vi "仁科参数读取.vi"() -> (2 "error out":errorcluster, 3 "簇":T1 {"时间 16"."分钟" format="%.0f分"; "时间 16"."小时" format="%.0f点"; "时间 15"."分钟" format="%.0f分"; "时间 15"."小时" format="%.0f点"; "时间 14"."分钟" format="%.0f分"; "时间 14"."小时" format="%.0f点"; "时间 13"."分钟" format="%.0f分"; "时间 13"."小时" format="%.0f点"; "时间 12"."分钟" format="%.0f分"; "时间 12"."小时" format="%.0f点"; "时间 11"."分钟" format="%.0f分"; "时间 11"."小时" format="%.0f点"; "时间 10"."分钟" format="%.0f分"; "时间 10"."小时" format="%.0f点"; "时间 9"."分钟" format="%.0f分"; "时间 9"."小时" format="%.0f点"; "时间 8"."分钟" format="%.0f分"; "时间 8"."小时" format="%.0f点"; "时间 7"."分钟" format="%.0f分"; "时间 7"."小时" format="%.0f点"; "时间 6"."分钟" format="%.0f分"; "时间 6"."小时" format="%.0f点"; "时间 5"."分钟" format="%.0f分"; "时间 5"."小时" format="%.0f点"; "时间 4"."分钟" format="%.0f分"; "时间 4"."小时" format="%.0f点"; "时间 3"."分钟" format="%.0f分"; "时间 3"."小时" format="%.0f点"; "时间 2"."分钟" format="%.0f分"; "时间 2"."小时" format="%.0f点"; "时间"."分钟" format="%.0f分"; "时间"."小时" format="%.0f点"})   [LabVIEW 2016, in "环境动力监测库.lvlib" / "空调库.lvlib"]
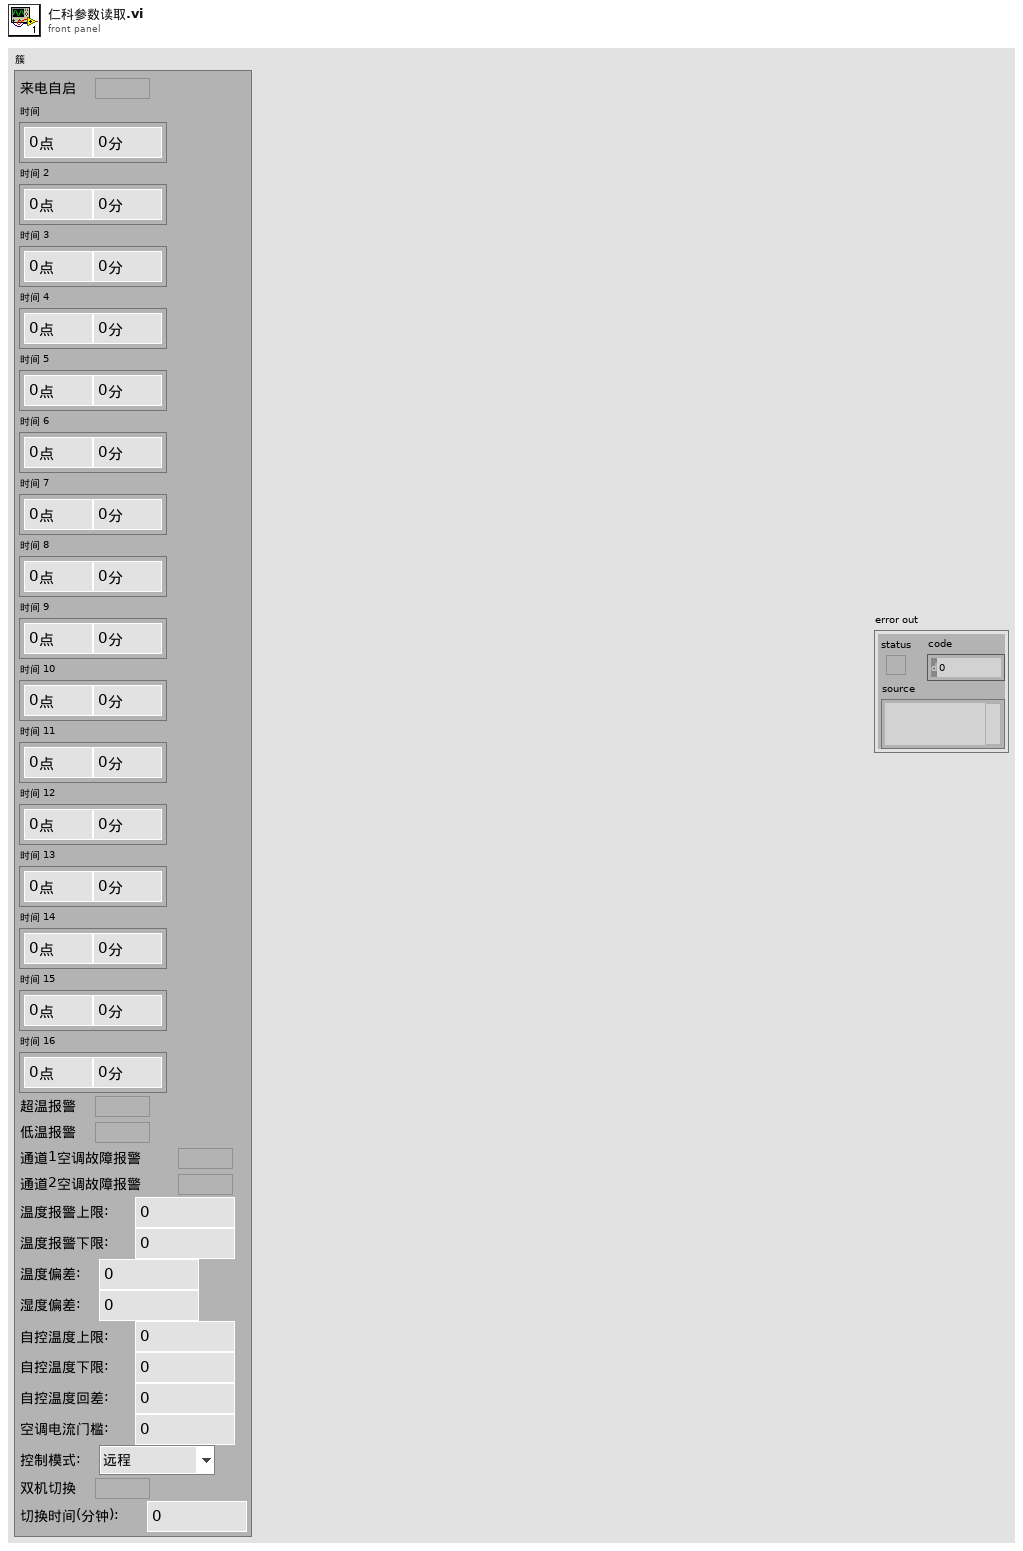
[diagram p1: front panel]
types:
  T1 = cluster{"来电自启":bool, "时间":cluster{"小时":u16, "分钟":u16}, "时间 2":cluster{"小时":u16, "分钟":u16}, "时间 3":cluster{"小时":u16, "分钟":u16}, "时间 4":cluster{"小时":u16, "分钟":u16}, "时间 5":cluster{"小时":u16, "分钟":u16}, "时间 6":cluster{"小时":u16, "分钟":u16}, "时间 7":cluster{"小时":u16, "分钟":u16}, "时间 8":cluster{"小时":u16, "分钟":u16}, "时间 9":cluster{"小时":u16, "分钟":u16}, "时间 10":cluster{"小时":u16, "分钟":u16}, "时间 11":cluster{"小时":u16, "分钟":u16}, "时间 12":cluster{"小时":u16, "分钟":u16}, "时间 13":cluster{"小时":u16, "分钟":u16}, "时间 14":cluster{"小时":u16, "分钟":u16}, "时间 15":cluster{"小时":u16, "分钟":u16}, "时间 16":cluster{"小时":u16, "分钟":u16}, "超温报警":bool, "低温报警":bool, "通道1空调故障报警":bool, "通道2空调故障报警":bool, "温度报警上限:":dbl, "温度报警下限:":dbl, "温度偏差:":dbl, "湿度偏差:":dbl, "自控温度上限:":dbl, "自控温度下限:":dbl, "自控温度回差:":dbl, "空调电流门槛:":dbl, "控制模式:":enum16{"远程", "自动"}, "双机切换":bool, "切换时间(分钟):":dbl}
  T2 = enum16{"open", "read", "write single", "write", "close"}
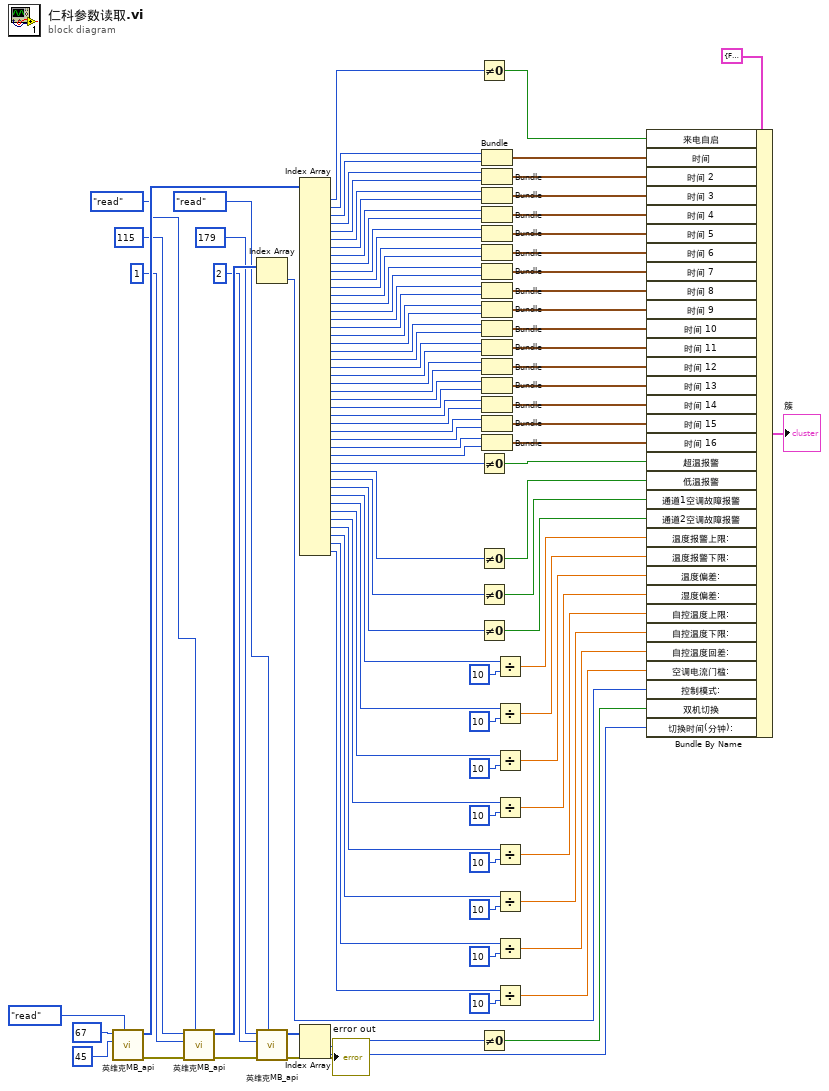
[diagram p0: block diagram]
diagram:
  n1 = call "英维克MB_api.vi"("STEP"=T2."read", "quantity"=u16 45, "starting address"=u16 67) -> ("error out"=w14:errorcluster, "Registers"=w100:u16[])  [unwired: 6 in, 1 out]
  n2 = call "英维克MB_api.vi"("STEP"=T2."read", "Error in"=w14, "quantity"=u16 1, "starting address"=u16 115) -> ("error out"=w7:errorcluster, "Registers"=w13:u16[])  [unwired: 5 in, 1 out]
  n3 = Index Array(array=w13) -> (element=w12:u16)  [unwired: 1 in]
  n4 = call "英维克MB_api.vi"("STEP"=T2."read", "Error in"=w7, "quantity"=u16 2, "starting address"=u16 179) -> ("error out"=→"error out":errorcluster, "Registers"=w11:u16[])  [unwired: 5 in, 1 out]
  n5 = Index Array(array=w100) -> (element #1=w99:u16, element #2=w98:u16, element #3=w97:u16, element #4=w96:u16, element #5=w95:u16, element #6=w91:u16, element #7=w90:u16, element #8=w89:u16, element #9=w88:u16, element #10=w85:u16, element #11=w84:u16, element #12=w83:u16, element #13=w82:u16, element #14=w79:u16, element #15=w78:u16, element #16=w77:u16, element #17=w76:u16, element #18=w75:u16, element #19=w74:u16, element #20=w73:u16, element #21=w72:u16, element #22=w71:u16, element #23=w70:u16, element #24=w69:u16, element #25=w68:u16, element #26=w61:u16, element #27=w60:u16, element #28=w59:u16, element #29=w58:u16, element #30=w57:u16, element #31=w56:u16, element #32=w55:u16, element #33=w54:u16, element #34=w49:u16, element #35=w48:u16, element #36=w47:u16, element #37=w46:u16, element #38=w41:u16, element #39=w37:u16, element #40=w34:u16, element #41=w31:u16, element #42=w26:u16, element #43=w25:u16, element #44=w24:u16, element #45=w19:u16)  [unwired: 45 in]
  n6 = Index Array(array=w11) -> (element #1=w6:u16, element #2=w4:u16)  [unwired: 2 in]
  n7 = Not Equal To 0?(x=w99) -> (x != 0?=w94:bool)
  n8 = Not Equal To 0?(x=w49) -> (x != 0?=w45:bool)
  n9 = Not Equal To 0?(x=w48) -> (x != 0?=w44:bool)
  n10 = Not Equal To 0?(x=w47) -> (x != 0?=w43:bool)
  n11 = Not Equal To 0?(x=w46) -> (x != 0?=w42:bool)
  n12 = Not Equal To 0?(x=w6) -> (x != 0?=w5:bool)
  n13 = Bundle(w98, w97) -> (w93:cluster{u16, u16})  [unwired: 1 in]
  n14 = Bundle(w96, w95) -> (w92:cluster{u16, u16})  [unwired: 1 in]
  n15 = Bundle(w91, w90) -> (w87:cluster{u16, u16})  [unwired: 1 in]
  n16 = Bundle(w89, w88) -> (w86:cluster{u16, u16})  [unwired: 1 in]
  n17 = Bundle(w85, w84) -> (w81:cluster{u16, u16})  [unwired: 1 in]
  n18 = Bundle(w83, w82) -> (w80:cluster{u16, u16})  [unwired: 1 in]
  n19 = Bundle(w79, w78) -> (w67:cluster{u16, u16})  [unwired: 1 in]
  n20 = Bundle(w77, w76) -> (w66:cluster{u16, u16})  [unwired: 1 in]
  n21 = Bundle(w75, w74) -> (w65:cluster{u16, u16})  [unwired: 1 in]
  n22 = Bundle(w73, w72) -> (w64:cluster{u16, u16})  [unwired: 1 in]
  n23 = Bundle(w71, w70) -> (w63:cluster{u16, u16})  [unwired: 1 in]
  n24 = Bundle(w69, w68) -> (w62:cluster{u16, u16})  [unwired: 1 in]
  n25 = Bundle(w61, w60) -> (w53:cluster{u16, u16})  [unwired: 1 in]
  n26 = Bundle(w59, w58) -> (w52:cluster{u16, u16})  [unwired: 1 in]
  n27 = Bundle(w57, w56) -> (w51:cluster{u16, u16})  [unwired: 1 in]
  n28 = Bundle(w55, w54) -> (w50:cluster{u16, u16})  [unwired: 1 in]
  n29 = Divide(x=w41, y=u16 10) -> (x/y=w39:dbl)
  n30 = Divide(x=w37, y=u16 10) -> (x/y=w36:dbl)
  n31 = Divide(x=w34, y=u16 10) -> (x/y=w33:dbl)
  n32 = Divide(x=w31, y=u16 10) -> (x/y=w30:dbl)
  n33 = Divide(x=w26, y=u16 10) -> (x/y=w23:dbl)
  n34 = Divide(x=w25, y=u16 10) -> (x/y=w22:dbl)
  n35 = Divide(x=w24, y=u16 10) -> (x/y=w21:dbl)
  n36 = Divide(x=w19, y=u16 10) -> (x/y=w18:dbl)
  n37 = Bundle By Name(cluster=T1 {"来电自启"=FALSE, "时间"={"小时"=0, "分钟"=0}, "时间 2"={"小时"=0, "分钟"=0}, "时间 3"={"小时"=0, "分钟"=0}, "时间 4"={"小时"=0, "分钟"=0}, "时间 5"={"小时"=0, "分钟"=0}, "时间 6"={"小时"=0, "分钟"=0}, "时间 7"={"小时"=0, "分钟"=0}, "时间 8"={"小时"=0, "分钟"=0}, "时间 9"={"小时"=0, "分钟"=0}, "时间 10"={"小时"=0, "分钟"=0}, "时间 11"={"小时"=0, "分钟"=0}, "时间 12"={"小时"=0, "分钟"=0}, "时间 13"={"小时"=0, "分钟"=0}, "时间 14"={"小时"=0, "分钟"=0}, "时间 15"={"小时"=0, "分钟"=0}, "时间 16"={"小时"=0, "分钟"=0}, "超温报警"=FALSE, "低温报警"=FALSE, "通道1空调故障报警"=FALSE, "通道2空调故障报警"=FALSE, "温度报警上限:"=0.0, "温度报警下限:"=0.0, "温度偏差:"=0.0, "湿度偏差:"=0.0, "自控温度上限:"=0.0, "自控温度下限:"=0.0, "自控温度回差:"=0.0, "空调电流门槛:"=0.0, "控制模式:"=enum."远程", "双机切换"=FALSE, "切换时间(分钟):"=0.0} ("簇"), "来电自启"=w94, "时间"=w93, "时间 2"=w92, "时间 3"=w87, "时间 4"=w86, "时间 5"=w81, "时间 6"=w80, "时间 7"=w67, "时间 8"=w66, "时间 9"=w65, "时间 10"=w64, "时间 11"=w63, "时间 12"=w62, "时间 13"=w53, "时间 14"=w52, "时间 15"=w51, "时间 16"=w50, "超温报警"=w45, "低温报警"=w44, "通道1空调故障报警"=w43, "通道2空调故障报警"=w42, "温度报警上限:"=w39, "温度报警下限:"=w36, "温度偏差:"=w33, "湿度偏差:"=w30, "自控温度上限:"=w23, "自控温度下限:"=w22, "自控温度回差:"=w21, "空调电流门槛:"=w18, "控制模式:"=w12, "双机切换"=w5, "切换时间(分钟):"=w4) -> (→"簇":T1)
